vi "ExtCall.vi"(8 "error in (no error)":errorcluster, 9 "Val":variant, 10 "Tag":u16, 11 "Rigol DG822 UI in":refnum<class "Rigol DG822 UI.lvclass">) -> (0 "error out":errorcluster, 1 "Response":variant, 3 "Rigol DG822 UI out":refnum<class "Rigol DG822 UI.lvclass">)   [LabVIEW 2021, in "Rigol DG822 UI.lvlib" / "Rigol DG822 UI.lvclass"]
uses:
  Rigol DG822 UI.lvclass
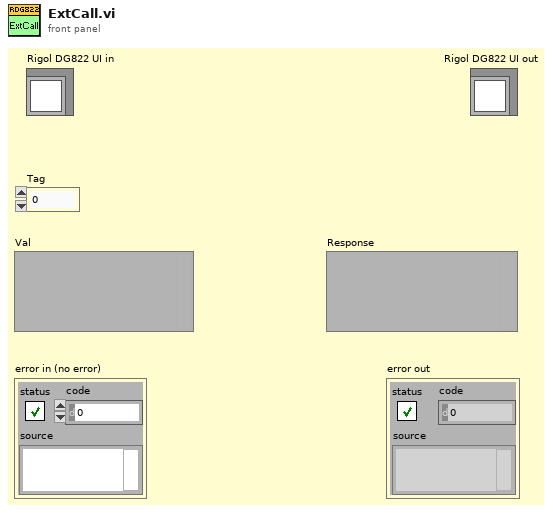
[diagram p1: front panel]
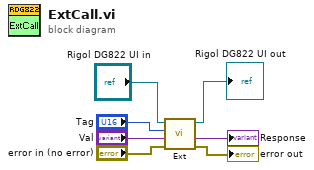
[diagram p0: block diagram]
diagram:
  n1 = call "Ext.vi"("error in (no error)"="error in (no error)", "Val"="Val", "Tag"="Tag", "Rigol DG822 UI in"="Rigol DG822 UI in") -> ("error out"=→"error out":errorcluster, "Parsed"=→"Response":variant, "Rigol DG822 UI out"=→"Rigol DG822 UI out":refnum<class "Rigol DG822 UI.lvclass">)  [unwired: 5 in]
